vi "MCP4725_with_GraphforLoopSingleArduinoInfiniteLoop.vi"() -> ()   [LabVIEW 2017]
uses:
  <vilib>/MakerHub/LINX/Public/Peripherals/Analog/Analog Read N Chans.vi
  <vilib>/MakerHub/LINX/Private/Local IO/LinxI2cWrite.vi
  <vilib>/MakerHub/LINX/Public/Utilities/Check Channel.vi
  <vilib>/MakerHub/LINX/Private/Local IO/LinxAnalogRead.vi
  <vilib>/MakerHub/LINX/Public/Utilities/Open Serial.vi
  <vilib>/MakerHub/LINX/Private/Utilties/Generate Error.vi
  <vilib>/Utility/file.llb/Write Delimited Spreadsheet (DBL).vi
  <vilib>/MakerHub/LINX/LMH-LINX.lvlib
panel:
  in  "?":bool
  in  "Save Data":bool
  out "XY Graph 2":cluster{dbl[], dbl[]}[](graph)
  out "XY Graph":cluster{dbl[], dbl[]}(graph)
  out "Voltage on Analog Channel":dbl(knob) scale=0.0..75.0
  out "Current Value written to \nDAC  input":u16
  out "Device Name":string
  out "Error Out":errorcluster
  in  "Data Collection\nTime  Interval (ms)":u32
  in  "Arduino \nSerial Port":refnum<visa-resource-name>="N/A"
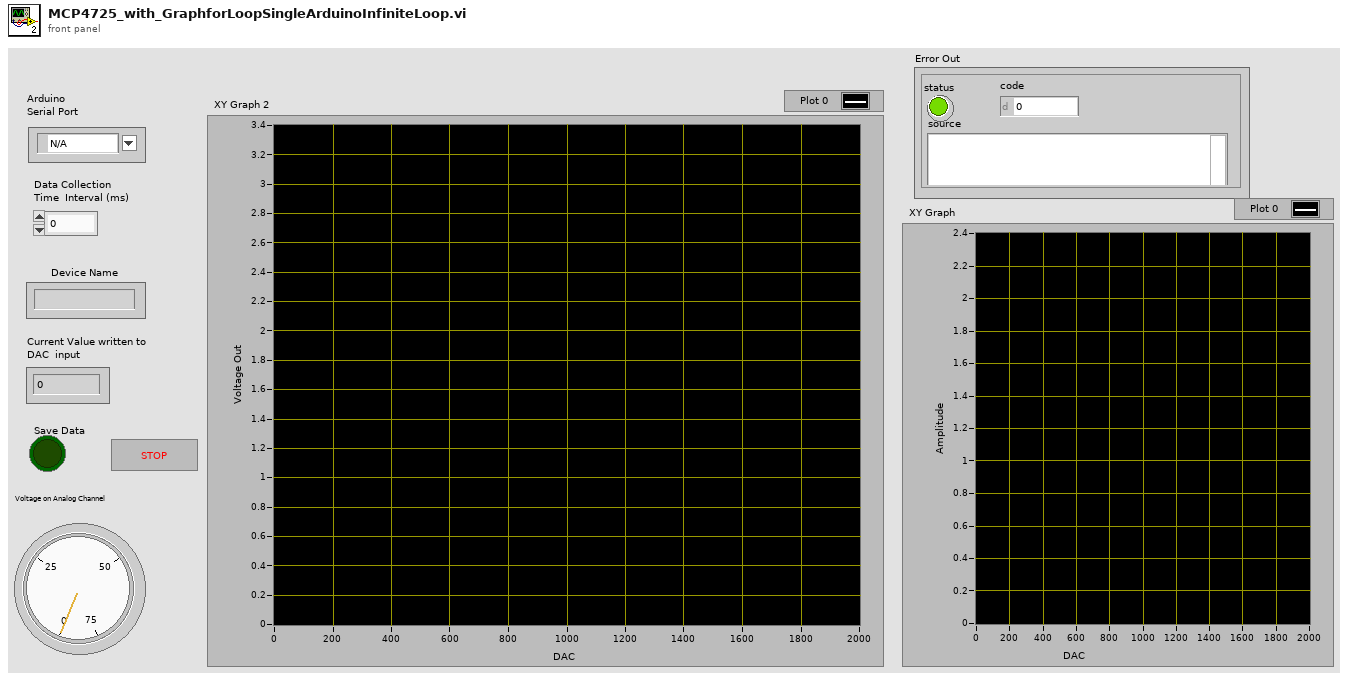
[diagram p1: front panel]
types:
  T1 = typedef "LMH-LINX.lvlib/LINX Ref.ctl" = cluster{"IO":T2, "Interface":T3, "LINX Device Config":T4}
  T2 = typedef "LMH-LINX.lvlib/Platform.ctl" = enum16{"Remote", "Local"}
  T3 = typedef "LMH-LINX.lvlib/Interface.ctl" = enum16{"Serial", "TCP"}
  T4 = typedef "LMH-LINX.lvlib/Device.lvlib/LINX Device Config.ctl" = cluster{"Interface":T3, "COM Port":refnum<visa-resource-name>, "TCP Configuration":T5, "Device Family":u8, "Device ID":u8, "Device Name":string, "TCP Ref":refnum<k5>, "Channels":T6}
  T5 = typedef "LMH-LINX.lvlib/Device.lvlib/TCP Config.ctl" = cluster{"IP Address":string, "Port":u16}
  T6 = typedef "LMH-LINX.lvlib/Channels.ctl" = cluster{"DI":u8[], "DO":u8[], "AI":u8[], "AO":u8[], "PWM":u8[], "QE":u8[], "UART":u8[], "I2C 2":u8[], "SPI":u8[], "CAN":u8[], "Servo":u8[], "AI Ref (V)":dbl, "AI Resolution (Bits)":u8, "AO Ref (V)":dbl, "AO Resolution (Bits)":u8}
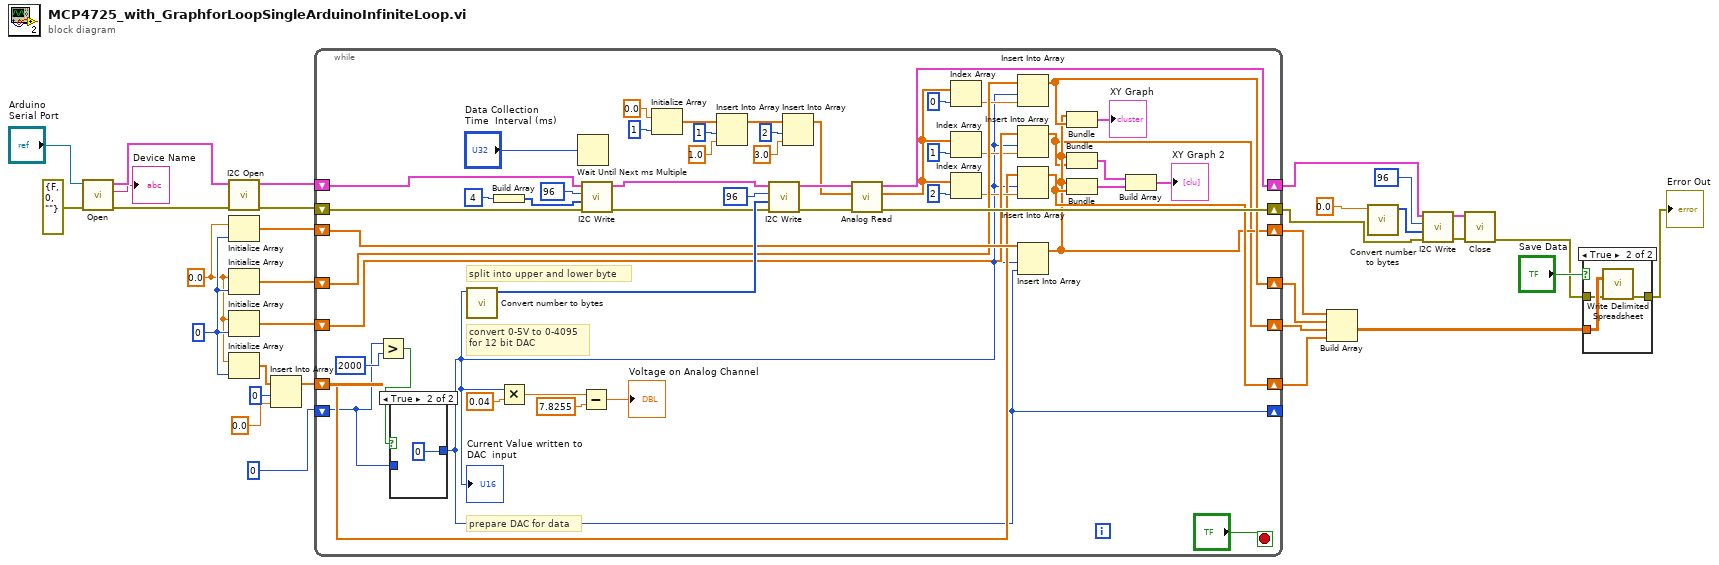
[diagram p0: block diagram]
diagram:
  w17 = 0.0 ("element")
  w18 = 0 ("dimension size")
  n1 = call-poly <vilib>:"Open.vi"("Error In"=errorcluster {"status"=FALSE, "code"=0, "source"=""}, "Serial Port"="Arduino \nSerial Port") -> ("Error Out"=w30:errorcluster, "Device Name"=→"Device Name":string, "LINX Resource"=w31:T1)  [unwired: 7 in]
  n2 = call <vilib>:"I2C Open.vi"("Error In"=w30, "LINX Resource"=w31) -> ("Error Out"=w27:errorcluster, "LINX Resource"=w28:T1)  [unwired: 8 in]
  n3 = Initialize Array(w17, w18) -> (w25:dbl[])
  n4 = Initialize Array(w17, w18) -> (w24:dbl[])
  n5 = Initialize Array(w17, w18) -> (w16:dbl[])
  n6 = Initialize Array(w17, w18) -> (w5:dbl[])
  n7 = Insert Into Array(array=w5, index=0, new element=0.0 ("new element/subarray")) -> (w2:dbl[])
  n8 = while {
    shift-right: [w74] -> w11
    shift-left: w28 -> [w83]
    shift-right: [w72] -> w8
    shift-left: w27 -> [w82]
    shift-right: [w46] -> w15
    shift-left: w25 -> [w70]
    shift-right: [w53] -> w14
    shift-left: w24 -> [w69]
    shift-right: [w45] -> w13
    shift-left: w16 -> [w52]
    shift-right: [w47] -> w12
    shift-left: w2 -> [w38]
    shift-right: [w33] -> _
    shift-left: 0 -> [w34]
    stop <- "?" stop-if-true
    # "prepare DAC for data"
    # "convert 0-5V to 0-4095\nfor 12 bit DAC"
    # "split into upper and lower byte"
    n9 = Greater?(x=w34, y=2000) -> (0:w36:bool)
    n10 = case shown="True" w36 {
      tunnel: [w84 0] -> w33
      tunnel: w34 -> [w84 _]
      frame False {
      }
      frame True {
      }
    }
    "Current Value written to \nDAC  input" <- w33
    n11 = call "Convert number to bytes.vi"("Numeric"=w33) -> ("Array"=w80:u8[])  [unwired: 10 in]
    n12 = Build Array(u8 4) -> (w76:u8[])
    n13 = Multiply(x=w33, y=0.04) -> (x*y=w56:dbl)
    n14 = Wait Until Next ms Multiple(millisecond multiple="Data Collection\nTime  Interval (ms)") -> ()  [unwired: 1 out]
    n15 = Subtract(x=w56, y=7.8255) -> (x-y=→"Voltage on Analog Channel":dbl)
    n16 = call <vilib>:"I2C Write.vi"("Error In"=w82, "Data"=w76, "I2C Slave Address (0)"=u8 96, "LINX Resource"=w83) -> ("Error Out"=w67:errorcluster, "LINX Resource"=w66:T1)  [unwired: 6 in]
    n17 = Initialize Array(0.0 ("element"), 1 ("dimension size")) -> (w63:dbl[])
    n18 = Insert Into Array(array=w63, index=1, new element=1.0 ("new element/subarray")) -> (w60:dbl[])
    n19 = call <vilib>:"I2C Write.vi"("Error In"=w67, "Data"=w80, "I2C Slave Address (0)"=u8 96, "LINX Resource"=w66) -> ("Error Out"=w73:errorcluster, "LINX Resource"=w75:T1)  [unwired: 6 in]
    n20 = Insert Into Array(array=w60, index=2, new element=3.0 ("new element/subarray")) -> (w57:dbl[])
    n21 = call-poly <vilib>:"Analog Read.vi"("Error In"=w73, "AI Channel(s)"=w57, "LINX Resource"=w75) -> ("Error Out"=w72:errorcluster, "Voltages"=w49:dbl[], "LINX Resource"=w74:T1)  [unwired: 5 in, 1 out]
    n22 = Index Array(array=w49, index=0) -> (element=w48:dbl)
    n23 = Index Array(array=w49, index=1) -> (element=w51:dbl)
    n24 = Index Array(array=w49, index=2) -> (element=w50:dbl)
    n25 = Insert Into Array(array=w69, index=w33, new element=w48) -> (w53:dbl[])
    n26 = Insert Into Array(array=w52, index=w33, new element=w51) -> (w45:dbl[])
    n27 = Insert Into Array(array=w38, index=w33, new element=w50) -> (w47:dbl[])
    n28 = Insert Into Array(array=w70, index=w33, new element=w33) -> (w46:dbl[])
    n29 = Bundle(w46, w53) -> (→"XY Graph":cluster{dbl[], dbl[]})  [unwired: 1 in]
    n30 = Bundle(w46, w45) -> (w43:cluster{dbl[], dbl[]})  [unwired: 1 in]
    n31 = Bundle(w46, w47) -> (w44:cluster{dbl[], dbl[]})  [unwired: 1 in]
    n32 = Build Array(w43, w44) -> (→"XY Graph 2":cluster{dbl[], dbl[]}[])
  }
  n33 = Build Array(w15, w14, w13, w12) -> (w10:dbl[][])
  n34 = call "Convert number to bytes.vi"("Numeric"=0.0) -> ("Array"=w22:u8[])  [unwired: 10 in]
  n35 = call <vilib>:"I2C Write.vi"("Error In"=w8, "Data"=w22, "I2C Slave Address (0)"=u8 96, "LINX Resource"=w11) -> ("Error Out"=w21:errorcluster, "LINX Resource"=w20:T1)  [unwired: 6 in]
  n36 = call <vilib>:"Close.vi"("Error In"=w21, "LINX Resource"=w20) -> ("Error Out"=w7:errorcluster)  [unwired: 9 in]
  n37 = case shown="True" "Save Data" {
    tunnel: [w86 w89] -> w6
    tunnel: w7 -> [w86 w87]
    tunnel: w10 -> [_ w88]
    frame False {
    }
    frame True {
      n38 = call-poly <vilib>:"Write Delimited Spreadsheet.vi"("2D data"=w88, "error in (no error)"=w87) -> ("error out"=w89:errorcluster)  [unwired: 12 in, 1 out]
    }
  }
  "Error Out" <- w6
